vi "GetItems.vi"(0 "VI Reference In":refnum<vi>, 5 "Control Path":string, 11 "error In":errorcluster) -> (4 "VI Reference Out":refnum<vi>, 6 "LstBox Refnum":refnum<vi>, 8 "Items[]":string[](array[string]), 15 "error out":errorcluster)   [LabVIEW 2020, in "ListBoxTests.lvlib"]
uses:
  ListBoxTests.lvlib
  <vilib>/SLL Drona/APIs/Get/GetControlRef/GetControlRefByPath.vi
  <vilib>/SLL Drona/Drona.lvlib
  <vilib>/SLL Drona/APIs/Get/GetControlRef/GetControlRef.lvlib
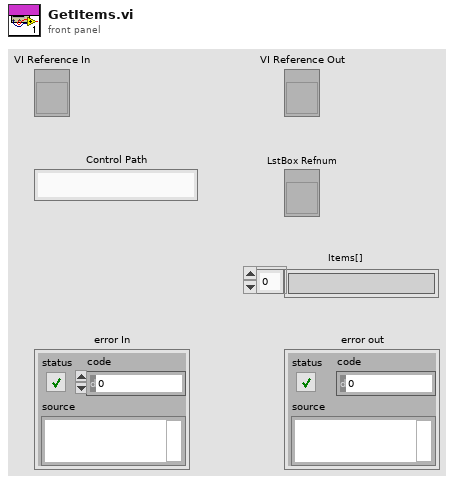
[diagram p1: front panel]
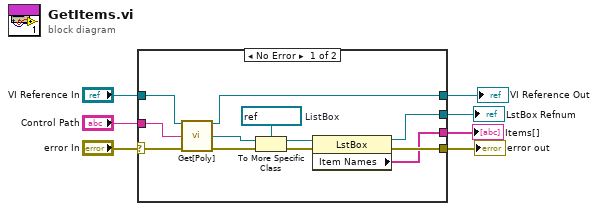
[diagram p0: block diagram]
diagram:
  n1 = case shown="No Error" "error In" {
    selector: "error In" -> [w17 w20]
    tunnel: "VI Reference In" -> [w19 w21]
    tunnel: "Control Path" -> [w18 _]
    tunnel: [w16 w21] -> w4
    tunnel: [w14 w20] -> w3
    tunnel: [w9 _] -> w2
    tunnel: [w8 _] -> w1
    frame No Error {
      w12 = refnum<vi> refnum  # ListBox
      n2 = call-poly <vilib>:"Get[Poly].vi"("VI Reference In"=w19, "Control Path"=w18, "error In"=w17) -> ("VI Reference Out"=w16:refnum<vi>, "Ctl Refnum"=w11:refnum<vi>, "error out"=w15:errorcluster)  [unwired: 10 in]
      n3 = To More Specific Class(target class=w12, reference=w11, error in=w15) -> (specific class reference=w10:refnum<vi>, error out=w13:errorcluster)
      n4 = property class="LstBox"(reference=w10, error in=w13) -> (reference out=w8:refnum<vi>, error out=w14:errorcluster, "Item Names"=w9:string[])
    }
    frame Error {
    }
  }
  "VI Reference Out" <- w4
  "error out" <- w3
  "Items[]" <- w2
  "LstBox Refnum" <- w1
